vi "Owl1553_BusControllerTransferBase_getTransferDescription.vi"(7 "error in (no error)":errorcluster, 10 "transferbase handle":u32) -> (0 "error out":errorcluster, 2 "transferdescription":string, 3 "transferbase handle":u32)   [LabVIEW 2014]
doc: "Gets the type of this transfer.\n\nReturns:\nOne of the TransferType enumeration values."
uses:
  <userlib>/MIL-STD-1553/Owl1553.lvlib
  owl1553.dll
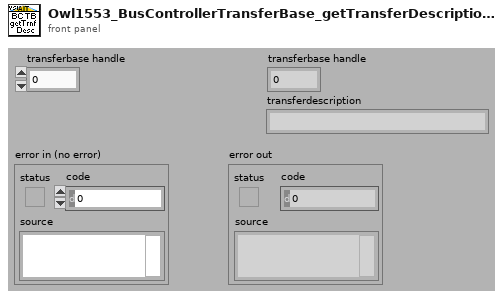
[diagram p1: front panel]
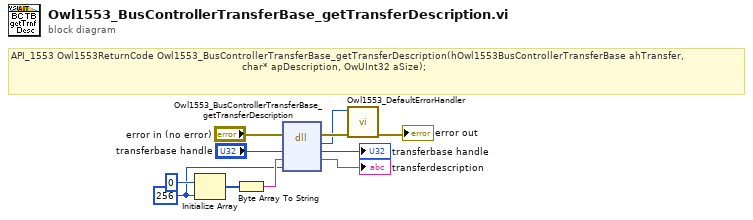
[diagram p0: block diagram]
diagram:
  w8 = 256 ("dimension size")
  # "API_1553 Owl1553ReturnCode Owl1553_BusControllerTransferBase_getTransferDescription(hOwl1553BusControllerTransferBase ahTransfer,\n                                                                             char* apDescription, OwUInt32 aSize);"
  n1 = Initialize Array(u8 0 ("element"), w8) -> (w11:u8[])
  n2 = Byte Array To String(unsigned byte array=w11) -> (string=w9:string)
  n3 = dll-call lib="owl1553.*" fn="Owl1553_BusControllerTransferBase_getTransferDescription" ("1553owl.*:Owl1553_BusControllerTransferBase_getTransferType")(error in="error in (no error)", "transferbase handle"="transferbase handle", "transferdescription"=w9, "size"=w8) -> (error out=w5:errorcluster, "return type"=w4:i32, "transferbase handle"=→"transferbase handle":u32, "transferdescription"=→"transferdescription":string)  [unwired: 3 in, 1 out]
  n4 = call <userlib>:"Owl1553_DefaultErrorHandler.vi"("error in (no error)"=w5, "error code"=w4) -> ("error out"=→"error out":errorcluster)  [unwired: 9 in]
